vi "Pendulum Read.vi"(11 "instance":i32) -> (3 "function return":i32)   [LabVIEW 2024, in "pendulumApp.lvlib"]
doc: "OOTB_API int Pendulum_Read(int instance);"
uses:
  pendulumApp.lvlib
  pendulumApp.dll
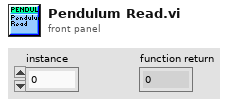
[diagram p1: front panel]
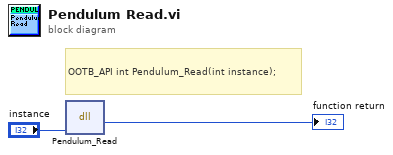
[diagram p0: block diagram]
diagram:
  # "OOTB_API\tint Pendulum_Read(int instance);"
  n1 = dll-call lib="C:/Users/scer/OneDrive - University of Florida/eml4314c/eml4314cFA25/Resources/FA25_dev_version2/SADI_Pendulum_lib/pendulumApp.*" fn="Pendulum_Read"("instance"="instance") -> (→"function return":i32)  [unwired: 4 in, 2 out]
